vi "Read Configuration File.vi"() -> (0 "Serial Numbers Found":bool, 5 "NI1":dbl, 7 "NI2":dbl)   [LabVIEW 2017]
uses:
  <vilib>/Utility/config.llb/Read Key (I32).vi
  <vilib>/Utility/config.llb/Read Key (String).vi
  <vilib>/Utility/config.llb/NI_LVConfig.lvlib
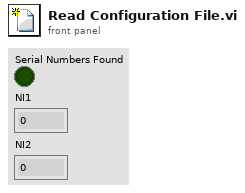
[diagram p1: front panel]
types:
  T1 = typedef "NI_LVConfig.lvlib/Config Data RefNum.ctl" = refnum<k1>
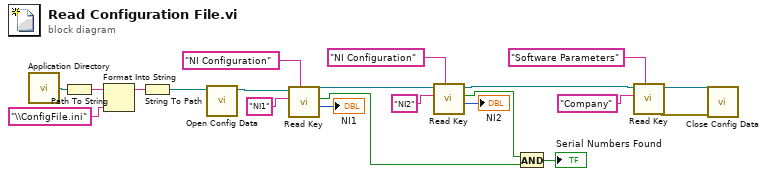
[diagram p0: block diagram]
diagram:
  n1 = call <vilib>:"Application Directory.vi"() -> ("Application Directory"=w21:path)
  n2 = Path To String(path=w21) -> (string=w20:string)
  n3 = Format Into String(initial string=w20, "\\ConfigFile.ini" ("string")) -> (resulting string=w18:string)  [unwired: 2 in, 1 out]
  n4 = String To Path(string=w18) -> (path=w17:path)
  n5 = call <vilib>:"Open Config Data.vi"("configuration file path"=w17) -> ("refnum"=w16:T1)  [unwired: 8 in, 2 out]
  n6 = call-poly <vilib>:"Read Key.vi"("section"="NI Configuration", "key"="NI1", "refnum"=w16) -> ("value"=→"NI1":i32, "found?"=w7:bool, "refnum out"=w11:T1)  [unwired: 5 in, 1 out]
  n7 = call-poly <vilib>:"Read Key.vi"("section"="NI Configuration", "key"="NI2", "refnum"=w11) -> ("value"=→"NI2":i32, "found?"=w8:bool, "refnum out"=w3:T1)  [unwired: 5 in, 1 out]
  n8 = And(x=w8, y=w7) -> (x .and. y?=→"Serial Numbers Found":bool)
  n9 = call-poly <vilib>:"Read Key.vi"("section"="Software Parameters", "key"="Company", "refnum"=w3) -> ("error out"=w1:errorcluster, "refnum out"=w2:T1)  [unwired: 5 in, 2 out]
  n10 = call <vilib>:"Close Config Data.vi"("error in (no error)"=w1, "refnum"=w2) -> ()  [unwired: 8 in, 2 out]
